vi "Nathan and Yasha Fail.vi"(9 "Current RPM":dbl) -> (1 "New RPM":dbl)   [LabVIEW 2012]
uses:
  Robot Global Data.vi
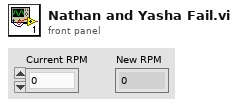
[diagram p1: front panel]
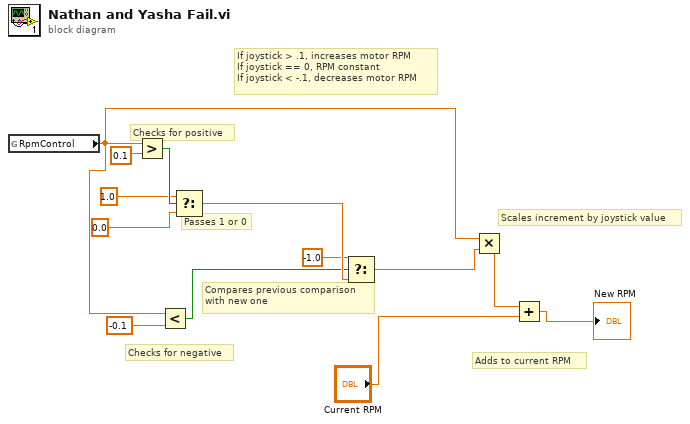
[diagram p0: block diagram]
diagram:
  # "If joystick > .1, increases motor RPM\nIf joystick == 0, RPM constant\nIf joystick < -.1, decreases motor RPM"
  # "Adds to current RPM"
  # "Scales increment by joystick value"
  # "Compares previous comparison\nwith new one"
  # "Checks for negative"
  # "Passes 1 or 0"
  # "Checks for positive"
  n1 = global read "Robot Global Data.vi" "RpmControl"() -> (w5:dbl)
  n2 = Greater?(x=w5, y=0.1) -> (0:w12:bool)
  n3 = Less?(x=w5, y=-0.1) -> (x < y?=w7:bool)
  n4 = Select(t=1.0, s=w12, f=0.0) -> (s? t:f=w9:dbl)
  n5 = Select(t=-1.0, s=w7, f=w9) -> (s? t:f=w4:dbl)
  n6 = Multiply(x=w5, y=w4) -> (x*y=w3:dbl)
  n7 = Add(x=w3, y="Current RPM") -> (x+y=→"New RPM":dbl)
